vi "dfd_IIR Filter Cluster Validation.vi"(8 "error in (no error)":errorcluster, 11 "IIR Filter Cluster":T1) -> (0 "error out":errorcluster, 3 "dup IIR Filter Cluster":T1)   [LabVIEW 2017, in "NI_DigFilterLicensed.lvlib"]
uses:
  <vilib>/addons/Digital Filter Design/NI_DigFilterLicensed.lvlib
  <vilib>/addons/Digital Filter Design/_Misc.llb/dfd_Error Handlers (Single).vi
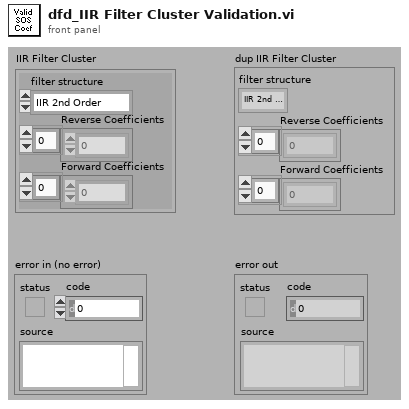
[diagram p1: front panel]
types:
  T1 = cluster{"filter structure":enum32{"IIR 2nd Order", "IIR 4th Order"}, "Reverse Coefficients":dbl[], "Forward Coefficients":dbl[]}
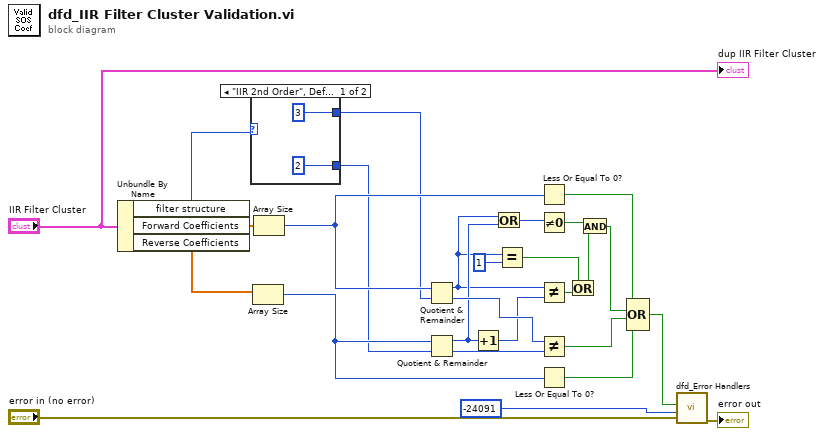
[diagram p0: block diagram]
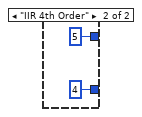
[diagram p2: hidden frame]
diagram:
  n1 = Unbundle By Name("IIR Filter Cluster") -> ("filter structure"=w3:enum32{"IIR 2nd Order", "IIR 4th Order"}, "Forward Coefficients"=w27:dbl[], "Reverse Coefficients"=w26:dbl[])
  n2 = case shown="\"IIR 2nd Order\", Default" w3 {
    tunnel: [3 ("y") 5 ("y")] -> w2
    tunnel: [2 ("y") 4 ("y")] -> w1
    frame "IIR 2nd Order", Default {
    }
    frame "IIR 4th Order" {
    }
  }
  n3 = Array Size(array=w26) -> (size(s)=w14:i32)
  n4 = Array Size(array=w27) -> (size(s)=w15:i32)
  n5 = Quotient & Remainder(x=w15, y=w2) -> (x-y*floor(x/y)=w6:i32, floor(x/y)=w22:i32)
  n6 = Quotient & Remainder(x=w14, y=w1) -> (x-y*floor(x/y)=w11:i32, floor(x/y)=w23:i32)
  n7 = Increment(x=w11) -> (x+1=w13:i32)
  n8 = Or(x=w6, y=w11) -> (x .or. y?=w10:i32)
  n9 = Equal?(x=w6, y=1) -> (x = y?=w4:bool)
  n10 = Less Or Equal To 0?(x=w15) -> (x <= 0?=w25:bool)
  n11 = Not Equal To 0?(x=w10) -> (x != 0?=w7:bool)
  n12 = Not Equal?(x=w6, y=w13) -> (x != y?=w8:bool)
  n13 = Not Equal?(x=w22, y=w23) -> (x != y?=w21:bool)
  n14 = Less Or Equal To 0?(x=w14) -> (x <= 0?=w24:bool)
  n15 = Or(x=w4, y=w8) -> (x .or. y?=w9:bool)
  n16 = And(x=w7, y=w9) -> (x .and. y?=w12:bool)
  n17 = Compound Arithmetic op=OR(w25, w12, w21, w24) -> (w19:bool)
  n18 = call-poly <vilib>:"dfd_Error Handlers.vi"("error in (no error)"="error in (no error)", "error code"=-24091 ("ERR_INVALID_SOS_COEF"), "condition failed?"=w19) -> ("error out"=→"error out":errorcluster)  [unwired: 8 out]
  "dup IIR Filter Cluster" <- "IIR Filter Cluster"
